vi "cam_wheel_origin.vi"(7 "에러 입력":errorcluster, 10 "FPGA VI 참조 입력":refnum<k20>) -> (0 "에러 출력":errorcluster, 1 "거리":dbl=42.0, 2 "차체각도":dbl=-8.857999999999999, 3 "FPGA VI 참조 출력":refnum<k20>)   [LabVIEW 2019]
uses:
  <vilib>/Platform/TimedLoop/XDataNode/timing_clust.ctl
  <vilib>/Platform/TimedLoop/XDataNode/nitl_modes.ctl
  <vilib>/Platform/TimedLoop/XDataNode/wakeup.ctl
  <vilib>/myRIO/Instrument Drivers/Onboard IO/UART/typedef/VISA Configuration.ctl
  <vilib>/Utility/error.llb/Error Cluster From Error Code.vi
  <vilib>/rvi/errors/niLvFpgaAdjustHostInterfaceError.vi
  <vilib>/rvi/interface/nirviReadWriteControl/nirviReadWriteControl.xnode
  <vilib>/Platform/TimedLoop/XDataNode/XDataNode.xnode
  <vilib>/Platform/TimedLoop/XDataNode/XDNodeRunTimeDep.lvlib
  <vilib>/rvi/interface/Simulation/niFpgaSimulationCallBeginRW.vi
  NiFpgaLv.dll
  <vilib>/myRIO/Instrument Drivers/Onboard IO/UART/UART.lvlib
panel:
  in  "L_pwm_List":dbl[](array[numeric])=[7000.0, 7000.0, 5000.0]
  in  "R_pwm_List":dbl[](array[numeric])=[8000.0, 7000.0, 5750.0]
  out "A/DIO4 (Pin 19)":bool=TRUE
  out "input":string="264/42"
  out "렢라 인덱스":i32=2
  in  "timed 정지":bool
  out "왼쪽 원소":dbl=8600.0
  in  "Left":dbl[](array[numeric])=[2800.0, -379.347, 8600.0]
  in  "Right":dbl[](array[numeric])=[2800.0, 379.347, 8600.0]
  out "2번(불까지거리)":string="42"
  out "1번(x픽셀)":string="264"
  out "s? t:f":dbl
  out "회전수 i":i32=18803
  out "x > y?":bool
  out "타임아웃":i32=-1
  out "L_encoder":i32
  out "R_Encoder":i32
  out "L_이동 거리":dbl=3461.010282721004
  out "R_이동 거리":dbl=3551.845719880893
  out "mm/ms":dbl=0.2573241845889076
  # "7000 7000"
  # "나중에 삭제해야함"
  # "2800 -379.347 8600\n2800 379.347 8600"
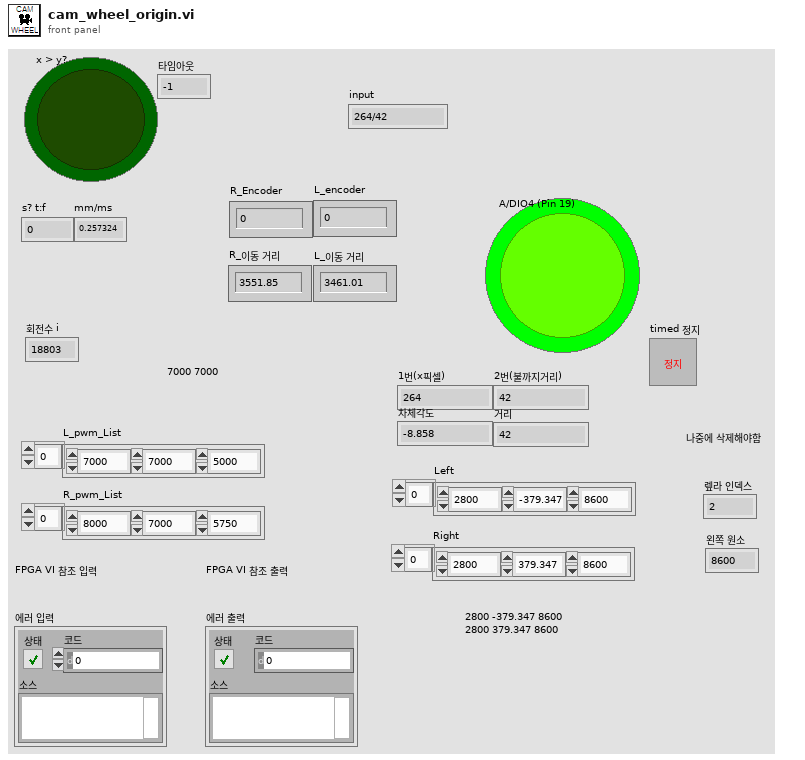
[diagram p1: front panel]
types:
  T1 = typedef "XDNodeRunTimeDep.lvlib/timing_clust.ctl" = cluster{"Expected End [f-1]":u64, "Actual End [f-1]":u64, "Finished Late? [f-1]":bool, "Expected End [i-1]":u64, "Actual End [i-1]":u64, "Finished Late? [i-1]":bool, "Expected Start [i]":u64, "Actual Start [i]":u64, "Expected Start [f]":u64, "Actual Start [f]":u64, "Source Name":string, "Structure Name":string, "Period":i64, "Deadline":i64, "Offset":i64, "Start":i64, "Priority":i32, "Timeout":i32, "Mode":T2, "Wakeup Reason":T3, "Error":errorcluster, "Source Type":string, "Secondary Source Type":string, "Global End Time":u64, "Global Start Time":u64, "Frame Duration":u64, "Iteration Duration":u64, "Assigned CPU":i32, "I/O Scan Engine Mode":u32}
  T2 = typedef "XDNodeRunTimeDep.lvlib/nitl_modes.ctl" = enum32{"No Change", "Process missed periods, maintain original phase", "Discard missed periods, maintain original phase", "Process missed periods, ignore original phase", "Discard missed periods, ignore original phase"}
  T3 = typedef "XDNodeRunTimeDep.lvlib/wakeup.ctl" = enum32{"Normal", "Aborted", "Asynchronous wakeup", "Timing source error", "Timed loop error", "Timeout"}
  T4 = typedef "UART.lvlib/VISA Configuration.ctl" = cluster{"baud rate (9600)":u32, "data bits (8)":u16, "parity (0:none)":enum16{"None", "Odd", "Even", "Mark", "Space"}, "stop bits (10: 1 bit)":u16, "flow control (0:none)":u16, "termination char\n(0xA = '\\n' = LF) ":u8, "Enable Termination\nChar (T)":bool, "timeout (10sec)":u32}
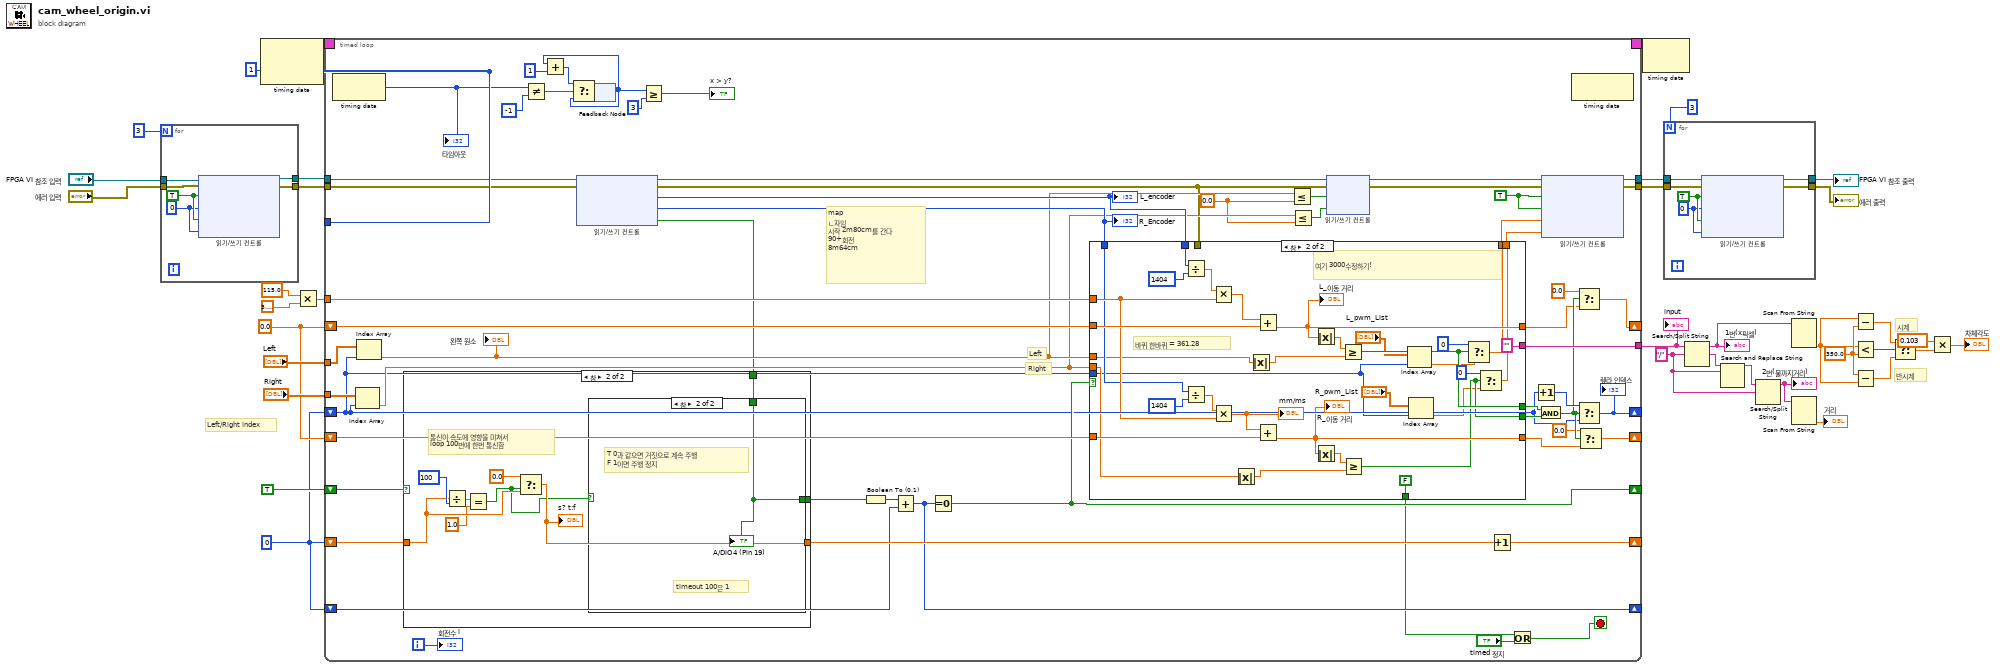
[diagram p0: block diagram]
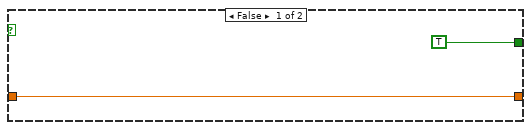
[diagram p2: hidden frame]
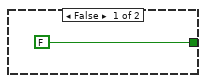
[diagram p3: hidden frame]
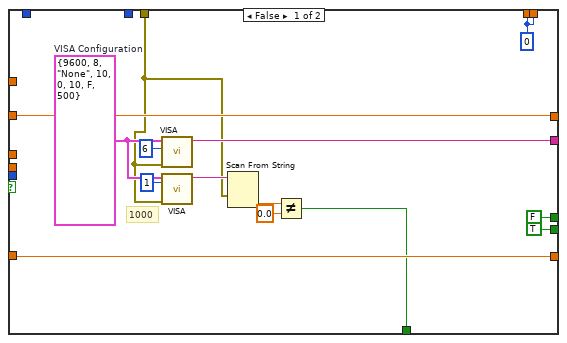
[diagram p4: hidden frame]
diagram:
  w8 = 350.0 ("y")
  w13 = 0.0
  w25 = "/" ("검색 문자열/문자 (-)")
  w12 = 0
  w27 = i64 1 ("주기")
  # "반시계"
  # "시계"
  # "Left/Right index"
  n1 = for {
    N: 3 -> [_]
    tunnel: [w42] -> w33
    tunnel: [w41] -> w32
    tunnel: "에러 입력" -> [w38]
    tunnel: "FPGA VI 참조 입력" -> [w37]
    w39 = 0 ("pwm input(escon)")
    w40 = TRUE ("encoder reset")
    n2 = xnode "읽기/쓰기 컨트롤"("FPGA VI 참조 입력"=w37, "에러 입력"=w38, "encoder reset"=w40, "pwm input"=w39, "R_encoder reset"=w40, "R_pwm input"=w39) -> ("FPGA VI 참조 출력"=w42:refnum<k20>, "에러 출력"=w41:errorcluster)
  }
  n3 = node-c288(w27) -> (w36:T1)  [unwired: 1 in]
  n4 = Multiply(x=115.0, y=3.141592653589793) -> (x*y=w28:dbl)
  n5 = timed-loop {
    timing: w36 -> [_]
    timing-out: [_] -> w35
    tunnel: w33 -> [w46]
    tunnel: w32 -> [w45]
    tunnel: [w92] -> w3
    tunnel: [w91] -> w2
    tunnel: w28 -> [w84]
    tunnel: w27 -> [_]
    shift-right: [w53] -> _
    shift-left: w13 -> [w85]
    shift-right: [w54] -> _
    shift-left: w13 -> [w86]
    shift-right: [w78] -> _
    shift-left: w12 -> [w76]
    shift-right: [w72] -> _
    shift-left: w12 -> [w73]
    shift-right: [w70] -> _
    shift-left: TRUE -> [w71]
    tunnel: [w69] -> w1
    tunnel: "Left" -> [w68]
    tunnel: "Right" -> [w67]
    shift-right: [w66] -> _
    shift-left: w12 -> [w43]
    i -> [w79]
    stop <- w55 stop-if-true
    w58 = 0.0 ("y")
    w90 = TRUE ("encoder reset")
    # "Right"
    # "Left"
    # "map\nㄴ자임\n시작 2m80cm를 간다\n90+회전\n8m64cm"
    n6 = node-c288() -> (w101:i32)  [unwired: 1 in]
    "타임아웃" <- w101
    n7 = Index Array(array=w67, index=w43) -> (element=w61:dbl)
    n8 = Index Array(array=w68, index=w43) -> (element=w62:dbl)
    "왼쪽 원소" <- w62
    n9 = Not Equal?(x=w101, y=-1) -> (x != y?=w99:bool)
    n10 = xnode "읽기/쓰기 컨트롤"("FPGA VI 참조 입력"=w46, "에러 입력"=w45) -> ("FPGA VI 참조 출력"=w88:refnum<k20>, "에러 출력"=w44:errorcluster, "Encoder  (4x)"=w83:i32, "R_Encoder  (4x)"=w82:i32, "camera"=w47:bool)
    "L_encoder" <- w83
    "R_Encoder" <- w82
    n11 = case shown="참" w71 {
      tunnel: [w102 w111] -> w77
      tunnel: w76 -> [w102 w109]
      tunnel: [TRUE w105] -> w74
      tunnel: w47 -> [_ w104]
      frame False {
      }
      frame True {
        # "통신이 속도에 영향을 미쳐서\nloop 100번에 한번 통신함"
        n12 = Divide(x=w109, y=100) -> (x/y=w108:dbl)
        n13 = Equal?(x=w108, y=1.0) -> (x = y?=w106:bool)
        n14 = Select(t=0.0, s=w106, f=w109) -> (s? t:f=w111:dbl)
        "s? t:f" <- w111
        n15 = case shown="참" w106 {
          tunnel: [FALSE w114] -> w105
          tunnel: w104 -> [_ w114]
          frame False {
          }
          frame True {
            # "timeout 100은 1"
            # "T 0과 같으면 거짓으로 계속 주행\nF 1이면 주행 정지"
            "A/DIO4 (Pin 19)" <- w114
          }
        }
      }
    }
    n16 = feedback #1() -> (w95:u8)  [unwired: 1 in]
    n17 = Add(x=w95, y=u8 1) -> (x+y=w98:u8)
    n18 = Select(t=w98, s=w99, f=w95) -> (s? t:f=w97:u8)
    n19 = feedback-in #1(w97) -> ()
    n20 = Greater Or Equal?(x=w95, y=u8 3) -> (x >= y?=→"x > y?":bool)
    n21 = Boolean To (0,1)(Boolean=w74) -> (0, 1=w75:i16)
    n22 = Add(x=w75, y=w73) -> (x+y=w72:i32)
    n23 = Equal To 0?(x=w72) -> (x = 0?=w70:bool)
    n24 = case shown="참" w70 {
      tunnel: [w126 w160] -> w48
      tunnel: w86 -> [w127 w159]
      tunnel: w85 -> [w126 w158]
      tunnel: w84 -> [_ w157]
      tunnel: w83 -> [_ w156]
      tunnel: w82 -> [_ w155]
      tunnel: [w119 FALSE] -> w57
      tunnel: [w128 w146] -> w81
      tunnel: [w128 w143] -> w80
      tunnel: [w127 w142] -> w49
      tunnel: [w124 "" ("read buffer")] -> w69
      tunnel: w62 -> [_ w136]
      tunnel: w61 -> [_ w134]
      tunnel: [FALSE w139] -> w64
      tunnel: [TRUE w138] -> w63
      tunnel: w44 -> [w115 _]
      tunnel: w43 -> [_ w130]
      frame False {
        w118 = T4 {"baud rate (9600)"=9600, "data bits (8)"=8, "parity (0:none)"=enum."None", "stop bits (10: 1 bit)"=10, "flow control (0:none)"=0, "termination char\n(0xA = '\\n' = LF) "=10, "Enable Termination\nChar (T)"=FALSE, "timeout (10sec)"=500}  # VISA Configuration
        w128 = 0 ("L_pwm")
        # "1000"
        n25 = call "VISA.vi"("에러 입력(에러 없음)"=w115, "바이트 카운트"=u32 6, "VISA Configuration"=w118) -> ("read buffer"=w124:string)  [unwired: 7 in, 1 out]
        n26 = call "VISA.vi"("에러 입력(에러 없음)"=w115, "바이트 카운트"=u32 1, "VISA Configuration"=w118) -> ("read buffer"=w117:string)  [unwired: 7 in, 1 out]
        n27 = Scan From String(input string=w117, error in=w115) -> (output 1=w121:dbl)  [unwired: 3 in, 3 out]
        n28 = Not Equal?(x=w121, y=0.0) -> (x != y?=w119:bool)
      }
      frame True {
        # "바퀴 한바퀴 = 361.28"
        # "여기 3000수정하기!"
        n29 = Divide(x=w156, y=1404) -> (x/y=w152:dbl)
        n30 = Divide(x=w155, y=1404) -> (x/y=w148:dbl)
        n31 = Multiply(x=w152, y=w157) -> (x*y=w153:dbl)
        n32 = Multiply(x=w148, y=w157) -> (x*y=w149:dbl)
        "mm/ms" <- w149
        n33 = Absolute Value(x=w134) -> (abs(x)=w135:dbl)
        n34 = Absolute Value(x=w136) -> (abs(x)=w137:dbl)
        n35 = Add(x=w153, y=w158) -> (x+y=w160:dbl)
        "L_이동 거리" <- w160
        n36 = Add(x=w149, y=w159) -> (x+y=w142:dbl)
        "R_이동 거리" <- w142
        n37 = Absolute Value(x=w160) -> (abs(x)=w151:dbl)
        n38 = Absolute Value(x=w142) -> (abs(x)=w147:dbl)
        n39 = Greater Or Equal?(x=w151, y=w137) -> (x >= y?=w139:bool)
        n40 = Greater Or Equal?(x=w147, y=w135) -> (x >= y?=w138:bool)
        n41 = Index Array(array="L_pwm_List", index=w130) -> (element=w131:dbl)
        n42 = Index Array(array="R_pwm_List", index=w130) -> (element=w132:dbl)
        n43 = Select(t=0, s=w139, f=w131) -> (s? t:f=w146:dbl)
        n44 = Select(t=0, s=w138, f=w132) -> (s? t:f=w143:dbl)
      }
    }
    n45 = Less Or Equal?(x=w62, y=w58) -> (x <= y?=w60:bool)
    n46 = Less Or Equal?(x=w61, y=w58) -> (x <= y?=w59:bool)
    n47 = xnode "읽기/쓰기 컨트롤"("FPGA VI 참조 입력"=w88, "에러 입력"=w44, "L_dir"=w60, "R_dir"=w59) -> ("FPGA VI 참조 출력"=w89:refnum<k20>, "에러 출력"=w87:errorcluster)
    n48 = Increment(x=w77) -> (x+1=w78:dbl)
    n49 = Or(x=w57, y="timed 정지") -> (x .or. y?=w55:bool)
    n50 = Increment(x=w43) -> (x+1=w65:i32)
    n51 = And(x=w64, y=w63) -> (x .and. y?=w52:bool)
    n52 = xnode "읽기/쓰기 컨트롤"("FPGA VI 참조 입력"=w89, "에러 입력"=w87, "encoder reset"=w90, "R_encoder reset"=w90, "pwm input"=w81, "R_pwm input"=w80) -> ("FPGA VI 참조 출력"=w92:refnum<k20>, "에러 출력"=w91:errorcluster)
    n53 = node-c288() -> ()  [unwired: 1 in, 1 out]
    n54 = Select(t=0.0, s=w52, f=w48) -> (s? t:f=w53:dbl)
    n55 = Select(t=w65, s=w52, f=w43) -> (s? t:f=w66:i32)
    "렢라 인덱스" <- w66
    n56 = Select(t=0.0, s=w52, f=w49) -> (s? t:f=w54:dbl)
    "회전수 i" <- w79
  }
  "input" <- w1
  n57 = node-c288(w35) -> ()  [unwired: 1 out]
  n58 = for {
    N: 3 -> [_]
    tunnel: [w167] -> w20
    tunnel: [w166] -> w19
    tunnel: w3 -> [w165]
    tunnel: w2 -> [w164]
    w168 = 0 ("pwm input(escon)")
    w169 = TRUE ("encoder reset")
    n59 = xnode "읽기/쓰기 컨트롤"("FPGA VI 참조 입력"=w165, "에러 입력"=w164, "encoder reset"=w169, "pwm input"=w168, "R_encoder reset"=w169, "R_pwm input"=w168) -> ("FPGA VI 참조 출력"=w167:refnum<k20>, "에러 출력"=w166:errorcluster)
  }
  "FPGA VI 참조 출력" <- w20
  "에러 출력" <- w19
  n60 = Search/Split String(string=w1, search string/char (-)=w25) -> (substring before match=w18:string, match + rest of string=w24:string)  [unwired: 2 out]
  "1번(x픽셀)" <- w18
  n61 = Search and Replace String(input string=w24, search string=w25) -> (result string=w23:string)  [unwired: 1 in, 8 out]
  n62 = Search/Split String(string=w23, search string/char (-)=w25) -> (substring before match=w17:string)  [unwired: 3 out]
  "2번(불까지거리)" <- w17
  n63 = Scan From String(input string=w18) -> (output 1=w7:dbl)  [unwired: 4 in, 3 out]
  n64 = Scan From String(input string=w17) -> (output 1=→"거리":dbl)  [unwired: 4 in, 3 out]
  n65 = Subtract(x=w7, y=w8) -> (x-y=w10:dbl)
  n66 = Less?(x=w7, y=w8) -> (x < y?=w11:bool)
  n67 = Subtract(x=w8, y=w7) -> (x-y=w9:dbl)
  n68 = Select(t=w10, s=w11, f=w9) -> (s? t:f=w6:dbl)
  n69 = Multiply(x=0.103, y=w6) -> (x*y=→"차체각도":dbl)
